vi "Create Header JSON.vi"(10 "error in (no error)":errorcluster, 11 "alg":string) -> (2 "error out":errorcluster, 3 "Header JSON":string)   [LabVIEW 2020, in "JWT.lvlib" / "JWT.lvclass"]
uses:
  JWT.lvclass
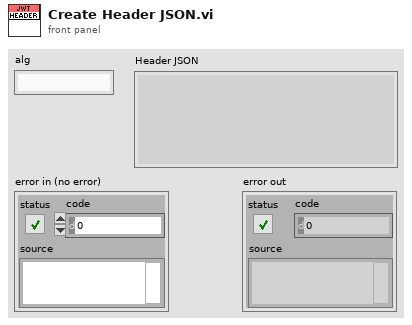
[diagram p1: front panel]
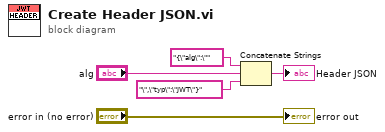
[diagram p0: block diagram]
diagram:
  n1 = Concatenate Strings("{\"alg\":\"" ("string"), "alg", "\",\"typ\":\"JWT\"}" ("string")) -> (→"Header JSON":string)
  "error out" <- "error in (no error)"
